vi "set_channel_offsets.vi"(8 "error in (no error)":errorcluster, 10 "pixel values cluster":T1, 11 "FPGAWrapperMH120124FrameScan_PXI7813R in":refnum<class "FPGAWrapperMH120124FrameScan_PXI7813R.lvclass">) -> (0 "error out":errorcluster, 3 "FPGAWrapperMH120124FrameScan_PXI7813R out":refnum<class "FPGAWrapperMH120124FrameScan_PXI7813R.lvclass">)   [LabVIEW 2010, in "FPGAWrapperMH120124FrameScan_PXI7813R.lvclass"]
uses:
  FPGAWrapperMH120124FrameScan_PXI7813R.lvclass
  common_typedefs/channels_cluster.ctl
  FPGAWrapperMH120124FrameScan_PXI7813R.lvclass/FPGAWrapperMH120124FrameScan_PXI7813R.ctl
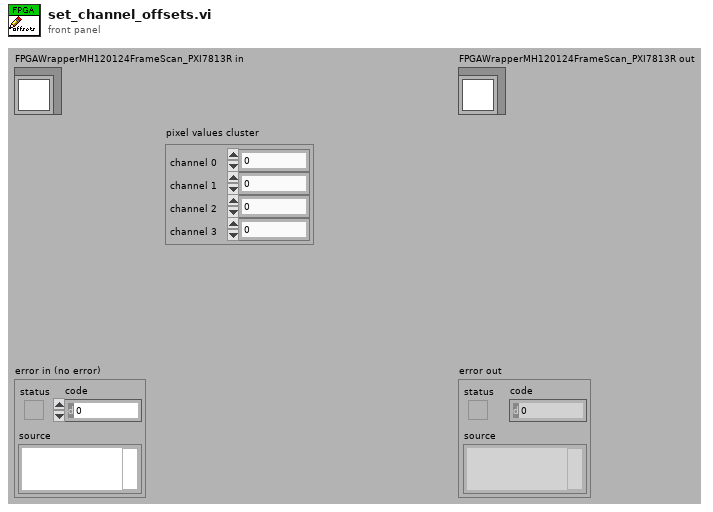
[diagram p1: front panel]
types:
  T1 = typedef "channels_cluster.ctl" = cluster{"channel 0":u32, "channel 1":u32, "channel 2":u32, "channel 3":u32}
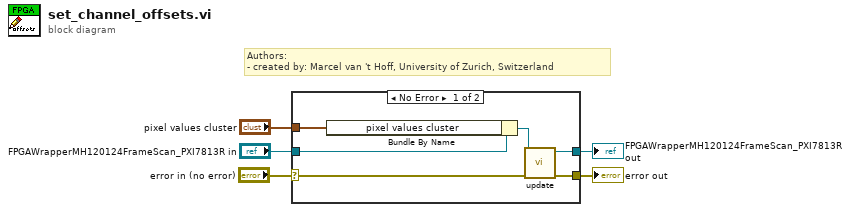
[diagram p0: block diagram]
diagram:
  # "Authors: \n- created by: Marcel van 't Hoff, University of Zurich, Switzerland"
  n1 = case shown="No Error" "error in (no error)" {
    selector: "error in (no error)" -> [w9 w13]
    tunnel: [w8 w13] -> w4
    tunnel: [w6 w12] -> w3
    tunnel: "FPGAWrapperMH120124FrameScan_PXI7813R in" -> [w11 w12]
    tunnel: "pixel values cluster" -> [w10 _]
    frame No Error {
      n2 = Bundle By Name(cluster=w11, "pixel values cluster"=w10) -> (w7:refnum<class "FPGAWrapperMH120124FrameScan_PXI7813R.lvclass">)
      n3 = call-dynamic "update.vi"("error in (no error)"=w9, "FPGAWrapperMH120124FrameScan_PXI7813R in"=w7) -> ("error out"=w8:errorcluster, "FPGAWrapperMH120124FrameScan_PXI7813R out"=w6:refnum<class "FPGAWrapperMH120124FrameScan_PXI7813R.lvclass">)  [unwired: 8 in]
    }
    frame Error {
    }
  }
  "error out" <- w4
  "FPGAWrapperMH120124FrameScan_PXI7813R out" <- w3
